vi "DS345_BurstMode.get ID.vi"(0 "i ref in":refnum<vi>, 5 "error in (no error)":errorcluster) -> (14 "i ref out":refnum<vi>, 15 "instrumentID":string, 19 "error out":errorcluster)   [LabVIEW 2014, in "DS345_BurstMode.lvlib"]
doc: "Reads the instrument ID string from the device."
uses:
  DS345_BurstMode.lvlib
  CSCore/CSSystem/CoreDefs/CoreDefs.error_type.ctl
  CSCore/CSSystem/CoreLib/CoreLib.lvlib
  CSCore/CSApplicationBaseClasses/DeviceBase/DeviceBase.lvlib
  CSCore/CSApplicationBaseClasses/DeviceBase/DeviceBase.deviceState.ctl
  CSlibraries-extern/DimLVEvent/NodeMon-LV/LVNodeInfo/LVNodeInfo.lvlib
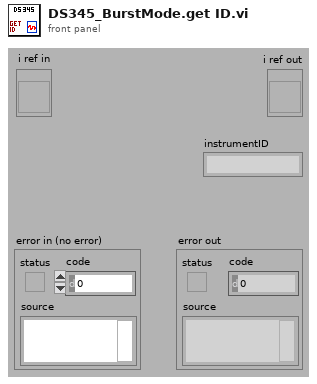
[diagram p1: front panel]
types:
  T1 = typedef "CoreDefs.error_type.ctl" = enum16{"no error", "can't load process", "can't unload process", "process does not exist", "can't install process", "can't remove process", "unknown function", "time out", "can't execute function", "duplicate queue name", "super not found", "caller queue invalid", "can't ping process", "unknown error", "VISA Error", "VISA timeout", "GPIB timeout", "GPIB error", "communication error", "data type mismatch", "can't read data from OPC server", "can't write data to OPC server", "OET error", "function not implemented", "process already exists", "invalid Shared Variable name", "error writing Shared Variable", "error reading Shared Variable", "invalid client name", "corrupt database", "unknown class", "call not authorized", "parameter out of range", "OET timeout: can't get data to modify", "invalid queue name", "requested operation incompatible with current state", "event undefined", "event disabled", "state undefined", "caller is not a friend", "EventBuilder: bad eventID", "EventBuilder: no DAQ devices", "a thread must not stop itself", "UNUSED ELEMENT4", "DiscArchiver: eventData incomplete", "DiscArchiver: eventData does not belong to run", "DiscArchiver: can't open file", "DiscArchiver: can't write to file", "DiscArchiver: available disc space low", "can't acquire semaphore", "error reading data from database", "notifier object is not existing", "can't register process", "can't unregister process", "illegal event type", "object disabled", "object already exists", "can't change state", "Instrument not found", "no connection to remote node", "invalid reference", "N/A", "UNUSED ELEMENT 1", "element not found", "illegal TCP/IP connection detected", "object does not exist", "invalid access ID", "unknown CS system", "invalid privilige", "unsupported data type", "unsupported server type", "IO server already exists", "Shared Variable already exists"}
  T2 = typedef "DeviceBase.lvlib/DeviceBase.deviceState.ctl" = i16
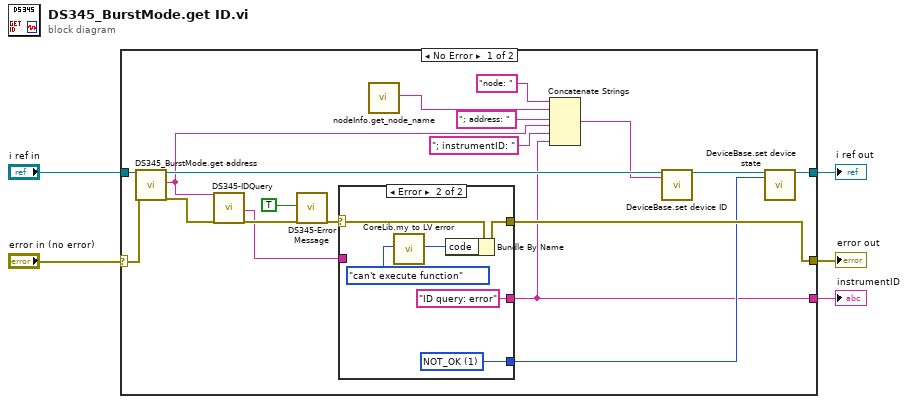
[diagram p0: block diagram]
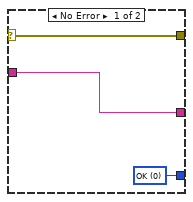
[diagram p2: hidden frame]
diagram:
  n1 = case shown="No Error" "error in (no error)" {
    selector: "error in (no error)" -> [w17 w34]
    tunnel: [w16 w34] -> w5
    tunnel: "i ref in" -> [w23 w35]
    tunnel: [w7 _] -> w3
    tunnel: [w14 w35] -> w2
    frame No Error {
      n2 = call "DS345_BurstMode.get address.vi"("i ref in"=w23, "error in (no error)"=w17) -> ("i ref out"=w18:refnum<vi>, "address"=w8:string, "error out"=w24:errorcluster)  [unwired: 15 in]
      n3 = call "DS345-IDQuery.vi"("GPIB in"=w8, "error in (no error)"=w24) -> ("instrumentID"=w19:string, "error out"=w22:errorcluster)  [unwired: 15 in, 1 out]
      n4 = call "DS345-Error Message.vi"("addMessageToSource"=TRUE ("add message to source"), "error in (no error)"=w22) -> ("error out"=w21:errorcluster)  [unwired: 14 in, 3 out]
      n5 = case shown="Error" w21 {
        selector: w21 -> [w27 w30]
        tunnel: [w27 w32] -> w16
        tunnel: [w26 "ID query: error" ("instrumentID")] -> w7
        tunnel: w19 -> [w26 _]
        tunnel: [w25 w29] -> w13
        frame No Error {
          w25 = T2 0 items=["ERROR"=-1, "OK"=0, "NOT_OK"=1] ("deviceState")
        }
        frame Error {
          w29 = T2 1 items=["ERROR"=-1, "OK"=0, "NOT_OK"=1] ("deviceState")
          n6 = call "CoreLib.my to LV error.vi"("ErrorTypes"=CoreDefs.error_type."can't execute function") -> ("LV error code"=w31:i32)  [unwired: 17 in, 1 out]
          n7 = Bundle By Name(cluster=w30, "code"=w31) -> (w32:errorcluster)
        }
      }
      n8 = call "nodeInfo.get_node_name.vi"() -> ("nodeName"=w9:string)  [unwired: 18 in, 1 out]
      n9 = Concatenate Strings("node: " ("string"), w9, "; address: " ("string"), w8, "; instrumentID: " ("string"), w7) -> (w6:string)
      n10 = call "DeviceBase.set device ID.vi"("i ref in"=w18, "deviceID"=w6) -> ("i ref out"=w15:refnum<vi>)  [unwired: 15 in, 2 out]
      n11 = call "DeviceBase.set device state.vi"("i ref in"=w15, "deviceState"=w13) -> ("i ref out"=w14:refnum<vi>)  [unwired: 15 in, 2 out]
    }
    frame Error {
    }
  }
  "error out" <- w5
  "i ref out" <- w2
  "instrumentID" <- w3
